vi "Init.vi"(3 "Container State":T5, 4 "Previous State":variant, 5 "Previous Version":T4) -> (2 "Current State":T1)   [LabVIEW 2017, in "UI_TimeSelector.xctl"]
uses:
  UI_TimeSelector.xctl
  State.ctl
  Typedefs/INTERNAL-DATA.ctl
  Interface/DEF-Mode.ctl
  <vilib>/_xctls/Container State.ctl
  <vilib>/_xctls/Version.ctl
  <vilib>/_xctls/XControlSupport.lvlib
panel:
  in  "Default Indicator State":T1
  in  "Default Control State":T1
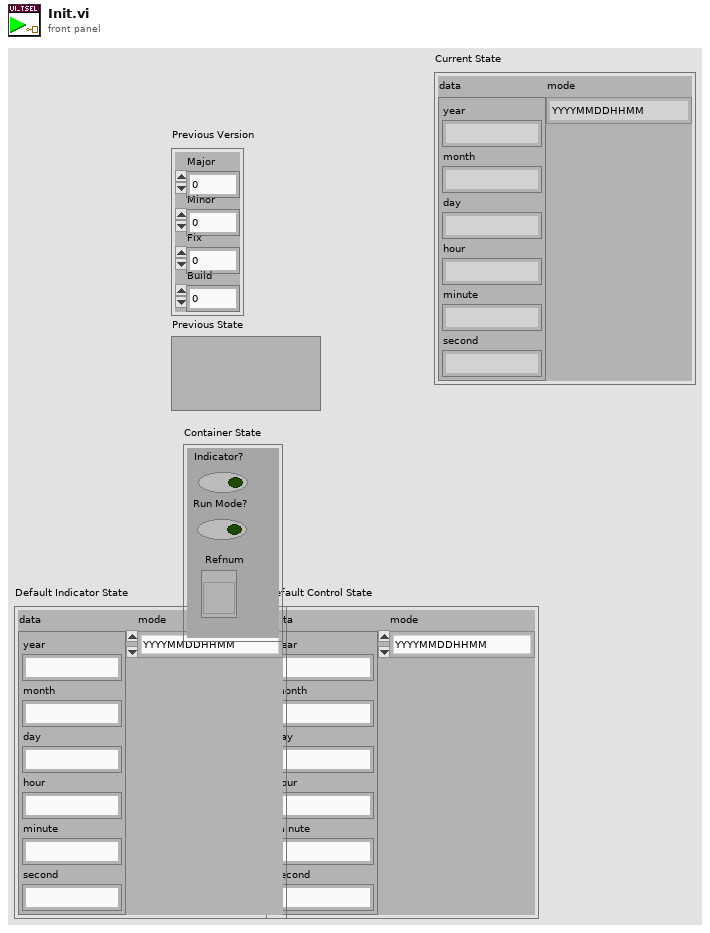
[diagram p1: front panel]
types:
  T1 = typedef "UI_TimeSelector.xctl/State.ctl" = cluster{"data":T2, "mode":T3}
  T2 = typedef "UI_TimeSelector.xctl/INTERNAL-DATA.ctl" = cluster{"year":string, "month":string, "day":string, "hour":string, "minute":string, "second":string}
  T3 = typedef "UI_TimeSelector.xctl/DEF-Mode.ctl" = enum16{"YYYYMMDDHHMM", "YYYYMMDDHHMMSS", "YYYY", "YYYYMM", "YYYYMMDD", "HHMM", "HHMMSS"}
  T4 = typedef "XControlSupport.lvlib/Version.ctl" = cluster{"Major":u16, "Minor":u16, "Fix":u16, "Build":u16}
  T5 = typedef "XControlSupport.lvlib/Container State.ctl" = cluster{"Indicator?":bool, "Run Mode?":bool, " Refnum":refnum<vi>}
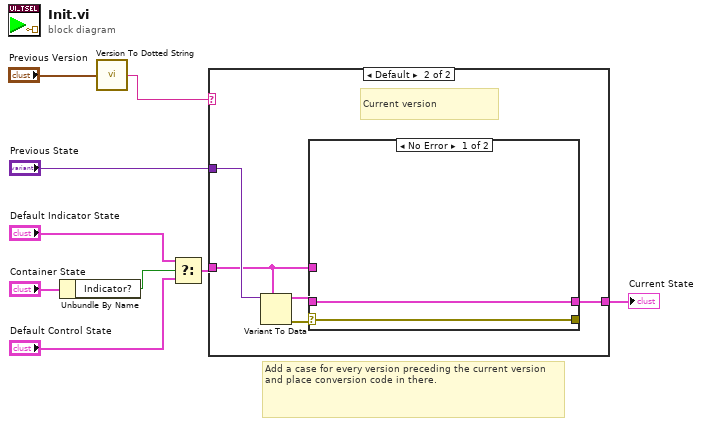
[diagram p0: block diagram]
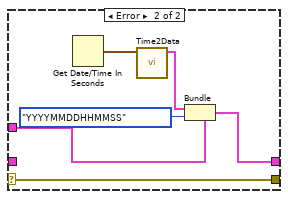
[diagram p3: hidden frame]
diagram:
  # "Add a case for every version preceding the current version and place conversion code in there."
  n1 = Unbundle By Name("Container State") -> ("Indicator?"=w4:bool)
  n2 = call <vilib>:"Version To Dotted String.vi"("Version"="Previous Version") -> ("String Version"=w1:string)
  n3 = Select(t="Default Indicator State", s=w4, f="Default Control State") -> (s? t:f=w3:T1)
  n4 = case shown="Default" w1 {
    tunnel: "Previous State" -> [_ w15]
    tunnel: [w10 w11] -> w8
    tunnel: w3 -> [w10 w12]
    frame "0.0.0.0" {
      # "Just created, use default state"
    }
    frame Default {
      # "Current version"
      n5 = Variant To Data(type=w12, Variant=w15) -> (data=w13:T1, error out=w14:errorcluster)  [unwired: 1 in]
      n6 = case shown="No Error" w14 {
        selector: w14 -> [w17 w23]
        tunnel: w13 -> [w16 _]
        tunnel: [w16 w21] -> w11
        tunnel: w12 -> [_ w22]
        tunnel: [w17 w23] -> _
        frame No Error {
        }
        frame Error {
          n7 = Get Date/Time In Seconds() -> (seconds since 1Jan1904=w20:timestamp)
          n8 = call "Time2Data.vi"("displayTime"=w20) -> ("data"=w19:T2)  [unwired: 10 in]
          n9 = Bundle(cluster=w22, "data"=w19, "mode"=DEF-Mode."YYYYMMDDHHMMSS") -> (w21:T1)
        }
      }
    }
  }
  "Current State" <- w8
